vi "AMWave.vi"() -> ()   [LabVIEW 2014]
panel:
  out "AM Wave":cluster{"Numeric":dbl}
  out "XY Graph":cluster{"X":dbl, "Y":dbl}[](graph)
  in  "Waveform Parameters":T1
  in  "Digitizing Parameters":T2
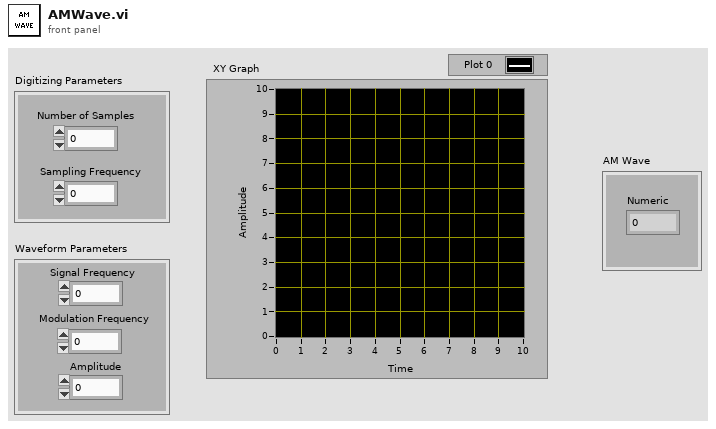
[diagram p1: front panel]
types:
  T1 = cluster{"Signal Frequency":dbl, "Modulation Frequency":dbl, "Amplitude":dbl}
  T2 = cluster{"Number of Samples":dbl, "Sampling Frequency":dbl}
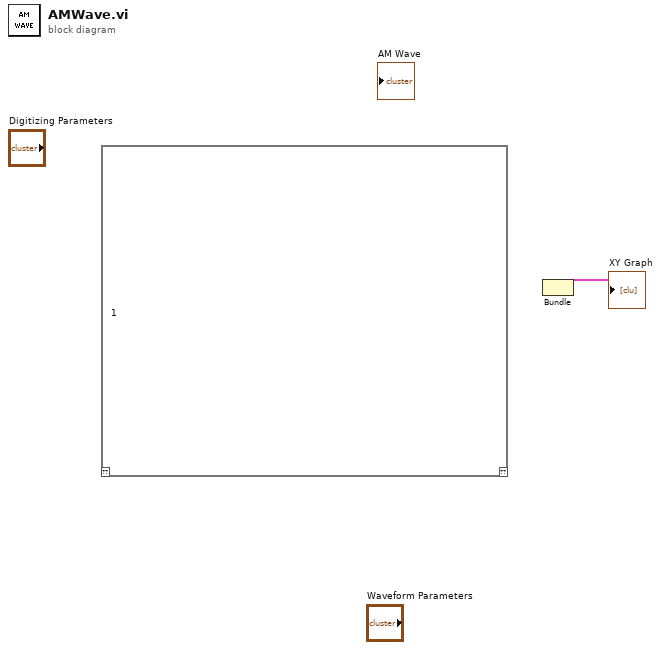
[diagram p0: block diagram]
diagram:
  n1 = mathscript code="1"() -> ()  [unwired: 1 in, 1 out]
  n2 = Bundle() -> (→"XY Graph":cluster{void, void})  [unwired: 3 in]
